vi "lib_QMH_Reset.vi"(8 "error in (no error)":errorcluster caption="错误输入（无错误）", 11 "Mod Admin in":refnum<class "lib_QMH_Module_Admin.lvclass">) -> (0 "error out":errorcluster caption="错误输出", 3 "Mod Admin out":refnum<class "lib_QMH_Module_Admin.lvclass">)   [LabVIEW 2018, in "lib_QMH_Module_Admin.lvclass"]
uses:
  lib_QMH_Module_Admin.lvclass
  lib_QMH_Module_Admin.lvclass/lib_QMH_Module_Admin.ctl
  lib_QMH_Set External Launch.vi
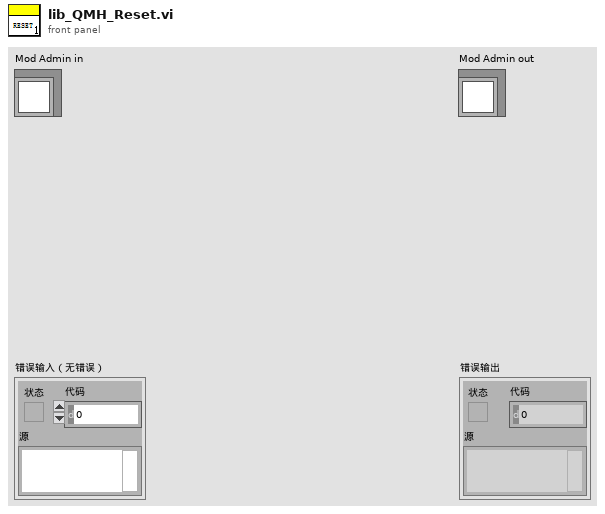
[diagram p1: front panel]
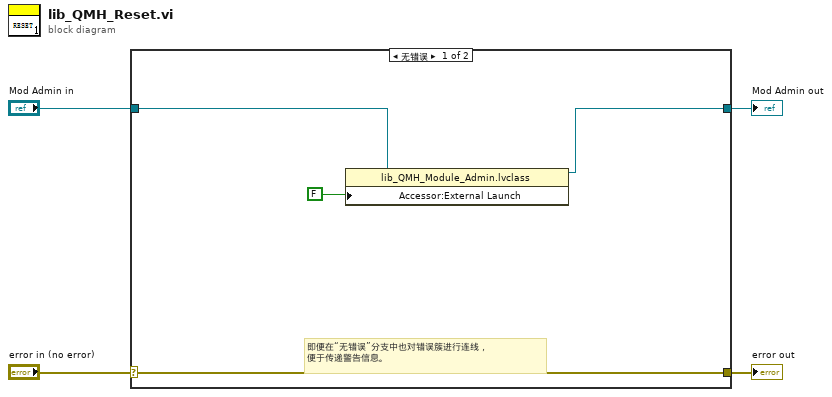
[diagram p0: block diagram]
diagram:
  n1 = case shown="无错误" "error in (no error)" {
    selector: "error in (no error)" -> [w8 w10]
    tunnel: [w8 w10] -> w3
    tunnel: [w5 w9] -> w1
    tunnel: "Mod Admin in" -> [w6 w9]
    frame No Error {
      # "即便在“无错误”分支中也对错误簇进行连线，\n便于传递警告信息。"
      n2 = property class="lib_QMH_Module_Admin.lvclass"(reference=w6, "Accessor:External Launch"=FALSE ("External Launch")) -> (reference out=w5:refnum<class "lib_QMH_Module_Admin.lvclass">)  [unwired: 1 in, 1 out]
    }
    frame Error {
    }
  }
  "error out" <- w3
  "Mod Admin out" <- w1
